vi "Flash APL Example.vi"(0 "Source Address":u8=228 format="%.0x", 5 "Destination Address":u8 format="%.0x", 7 "APL Path":path, 9 "Force Update?":bool, 11 "Error In":errorcluster) -> (4 "Result":T1(ring), 15 "Error Out":errorcluster)   [LabVIEW 2014, in "GEA2_Toolkit.lvlib"]
doc: "This standalone example will flash an APL file to the board specified."
uses:
  library/GEA2_Toolkit.lvlib
  Washer HCC/Washer HCC NEWFI/LabVIEW GEA2 Toolkit/LabVIEW_GEA2_Toolkit.lvlibp
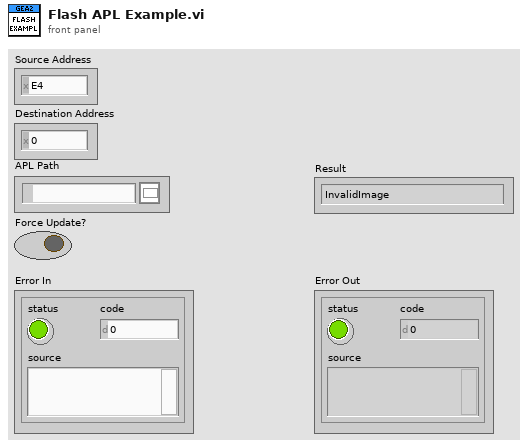
[diagram p1: front panel]
types:
  T1 = enum16{"InvalidImage", "ImageRejected", "BoardNotFound", "UnableToGetGeaConfiguration", "WriteToFlashNotAllowed", "ImageDownloadedSuccessfully", "ImagePresent", "WriteToFlashFailed", "EraseFailed", "CrcFailed"}
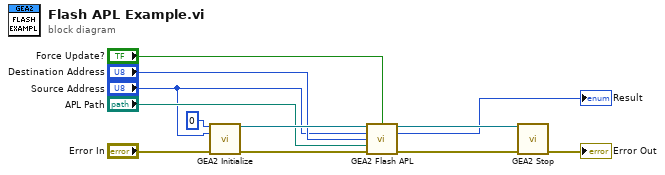
[diagram p0: block diagram]
diagram:
  n1 = call "GEA2 Initialize.vi"("Board Index"=0, "Source Address"="Source Address", "error in"="Error In") -> ("GEA2 Reference Out"=w12:refnum<k24>, "error out"=w11:errorcluster)  [unwired: 10 in, 1 out]
  n2 = call "GEA2 Flash APL.vi"("GEA2 Reference In"=w12, "Force Update?"="Force Update?", "Source Address"="Source Address", "Destination Address"="Destination Address", "File Path"="APL Path", "Error In"=w11) -> ("GEA2 Reference Out"=w8:refnum<k24>, "Result"=→"Result":i32, "Error Out"=w7:errorcluster)  [unwired: 7 in]
  n3 = call "GEA2 Stop.vi"("GEA2 Reference In"=w8, "Error In"=w7) -> ("Error Out"=→"Error Out":errorcluster)  [unwired: 13 in]
